vi "setControlTargetRange.vi"(8 "error":errorcluster, 9 "range":i32, 10 "axis":i32, 11 "connection ID":refnum<k5>) -> (0 "error out":errorcluster, 2 "axis_out":i32, 3 "connection ID out":refnum<k5>)   [LabVIEW 2016, in "amc_api.lvlib"]
doc: "This function sets the range around the target position in which the flag \"In Target Range\" (see VIII.7.a) becomes active."
uses:
  amc_api.lvlib
panel:
  out "jsonRespIn":string
  out "JSON-response":string="{\"jsonrpc\":\"2.0\",\"method\":\"\",\"params\":[5,1.245,true,\"name\"],\"id\":\"1\"}"
  out "JSON request":string
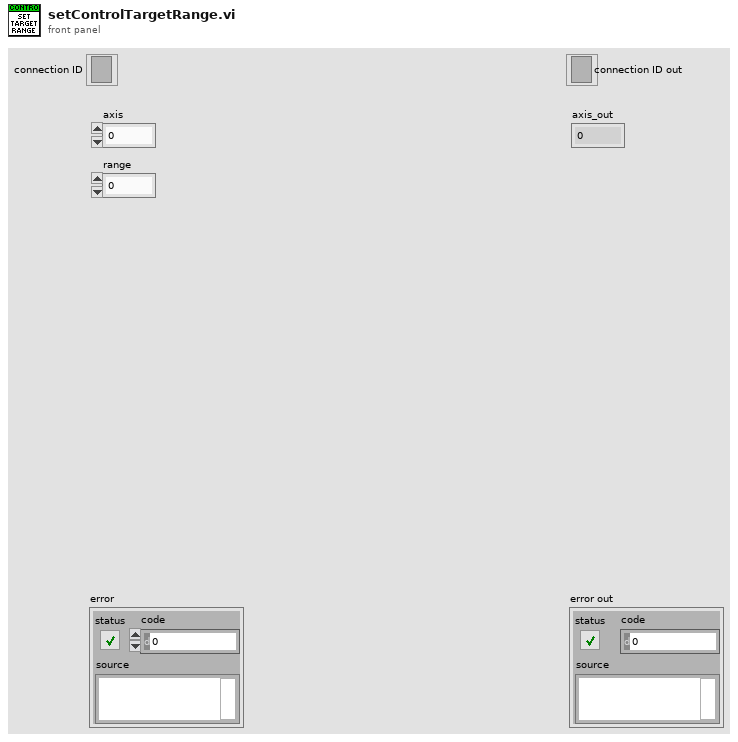
[diagram p1: front panel]
types:
  T1 = cluster{"jsonrpc":string, "method":string, "params":string[], "id":string, "api":i32, "pid":string}
  T2 = enum16{"Standard", "Buffered", "CRLF", "Immediate"}
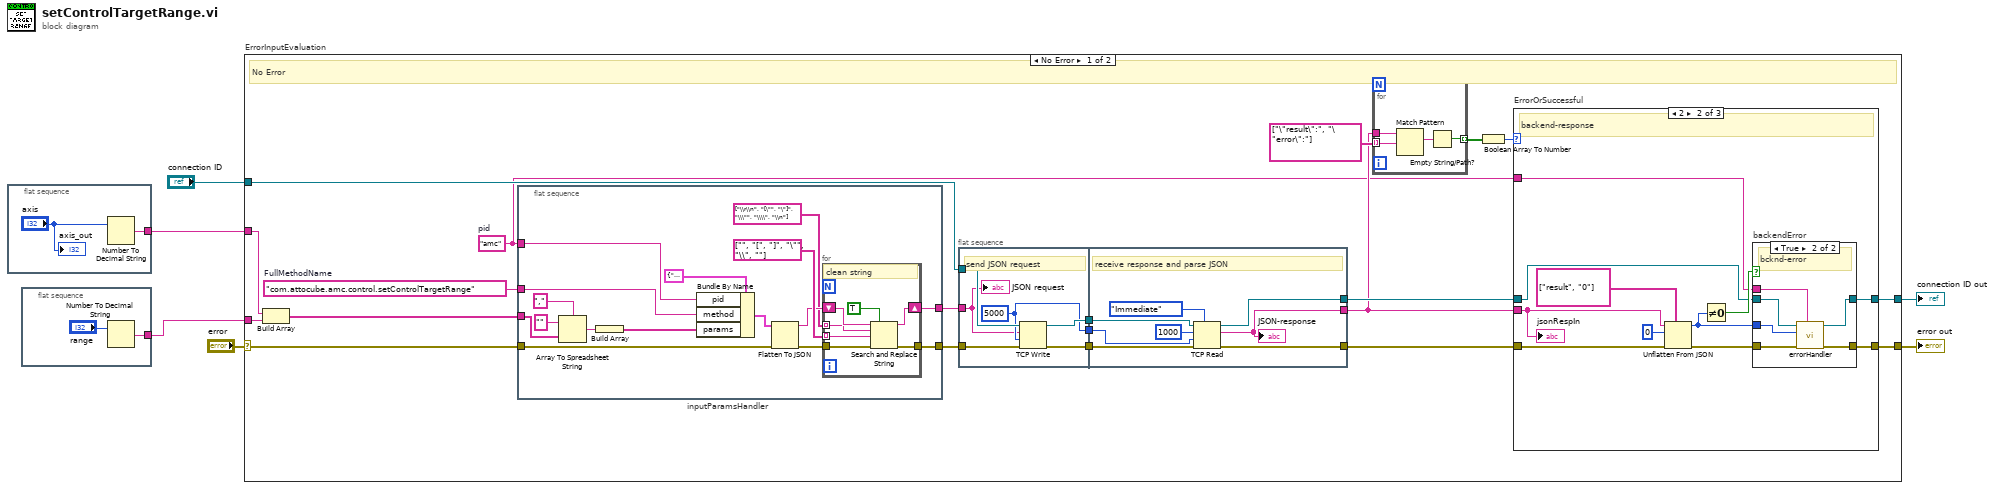
[diagram p0: block diagram]
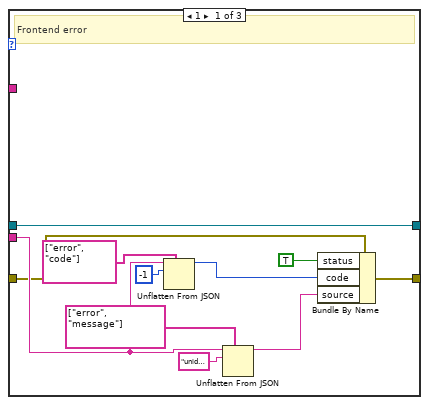
[diagram p2: hidden frame]
diagram:
  n1 = flat-sequence "in_axis" {
    tunnel: [w8] -> w2
    frame #0 {
      n2 = Number To Decimal String(number="axis") -> (decimal integer string=w8:string)  [unwired: 1 in]
      "axis_out" <- "axis"
    }
  }
  n3 = flat-sequence "in_integer" {
    tunnel: [w9] -> w1
    frame #0 {
      n4 = Number To Decimal String(number="range") -> (decimal integer string=w9:string)  [unwired: 1 in]
    }
  }
  n5 = case "ErrorInputEvaluation" shown="No Error" "error" {
    selector: "error" -> [w17 w104]
    tunnel: "connection ID" -> [w27 w105]
    tunnel: [w19 w104] -> w5
    tunnel: [w20 w105] -> w4
    tunnel: w2 -> [w12 _]
    tunnel: w1 -> [w11 _]
    frame No Error {
      w13 = "amc"  # pid
      w18 = "com.attocube.amc.control.setControlTargetRange"  # FullMethodName
      # "No Error"
      n6 = Build Array ("ParametersArrayString")(w12, w11) -> (w16:string[])
      n7 = flat-sequence "inputParamsHandler" {
        tunnel: [w36] -> w15
        tunnel: w16 -> [w42]
        tunnel: w17 -> [w41]
        tunnel: [w38] -> w14
        tunnel: w18 -> [w32]
        tunnel: w13 -> [w31]
        frame #0 {
          n8 = Array To Spreadsheet String(delimiter (Tab)=",", array=w42, 3:"" ("format string")) -> (spreadsheet string=w44:string)
          n9 = Build Array "Build Array"(w44) -> (w33:string[])
          n10 = Bundle By Name(cluster=T1 {"jsonrpc"="2.0", "method"="com.attocube.amc.res.setRESReadOutFreq", "params"=[], "id"="1", "api"=2, "pid"=""}, "pid"=w31, "method"=w32, "params"=w33) -> (w43:T1)
          n11 = Flatten To JSON(anything=w43, error in (no error)=w41) -> (JSON string=w37:string, 11:w39:errorcluster)  [unwired: 1 in]
          n12 = for {
            tunnel: string[] ["\\r\\n", "[\"", "\"]", "\\\"", "\\\\", "\\n"] ("search string") -> [w50] mode=indexing
            tunnel: string[] ["", "[", "]", "\"", "\\", ""] ("replace string (\"\")") -> [w49] mode=indexing
            shift-right: [w52] -> w36
            shift-left: w37 -> [w51]
            tunnel: w39 -> [w48]
            tunnel: [w47] -> w38
            # "clean string"
            n13 = Search and Replace String(replace all?=TRUE ("replace all? (F)"), input string=w51, search string=w50, replace string=w49, error in=w48) -> (result string=w52:string, error out=w47:errorcluster)  [unwired: 3 in, 2 out]
          }
        }
      }
      n14 = flat-sequence {
        tunnel: w27 -> [w95]
        tunnel: [w93] -> w30
        tunnel: [w94] -> w29
        tunnel: w14 -> [w90]
        tunnel: [w92] -> w28
        tunnel: w15 -> [w91]
        tunnel: [w99] -> w23
        tunnel: w30 -> [w101]
        tunnel: w29 -> [w100]
        tunnel: [w97] -> w22
        tunnel: w28 -> [w98]
        tunnel: [w96] -> w21
        frame #0 {
          w92 = 5000 ("timeout ms (25000)")
          # "send JSON request"
          n15 = TCP Write(connection ID=w95, data in=w91, error in (no error)=w90, 9:w92) -> (connection ID out=w93:refnum<k5>, error out=w94:errorcluster)  [unwired: 1 out]
          "JSON request" <- w91
        }
        frame #1 {
          # "receive response and parse JSON"
          n16 = TCP Read(connection ID=w101, bytes to read=1000, error in (no error)=w100, 7:T2."Immediate" ("mode (standard)"), 9:w98) -> (connection ID out=w99:refnum<k5>, data out=w96:string, error out=w97:errorcluster)
          "JSON-response" <- w96
        }
      }
      n17 = for {
        tunnel: string[] ["\"result\":", "\"error\":"] ("path") -> [w56] mode=indexing
        tunnel: [w54] -> w25 mode=indexing
        tunnel: w21 -> [w57]
        n18 = Match Pattern(string=w57, regular expression=w56) -> (match substring=w55:string)  [unwired: 1 in, 3 out]
        n19 = Empty String/Path?(string/path=w55) -> (empty?=w54:bool)
      }
      n20 = Boolean Array To Number(Boolean array=w25) -> (number=w24:u32)
      n21 = case "ErrorOrSuccessful" shown="2" w24 {
        tunnel: w21 -> [w60 w70 _]
        tunnel: w23 -> [w58 w73 w89]
        tunnel: [w58 w72 w89] -> w20
        tunnel: [w61 w71 w88] -> w19
        tunnel: w22 -> [w59 w74 w88]
        tunnel: w13 -> [_ w69 _]
        frame 1 {
          # "Frontend error"
          n22 = Unflatten From JSON(path=string[] ["error", "code"], JSON string=w60, type and defaults=-1) -> (value=w67:i32)  [unwired: 4 in, 1 out]
          n23 = Unflatten From JSON(path=string[] ["error", "message"], JSON string=w60, type and defaults="unidentified error") -> (value=w68:string)  [unwired: 4 in, 1 out]
          n24 = Bundle By Name(cluster=w59, "status"=TRUE, "code"=w67, "source"=w68) -> (w61:errorcluster)
        }
        frame 2 {
          # "backend-response"
          n25 = Unflatten From JSON(path=string[] ["result", "0"], JSON string=w70, type and defaults=0, error in (no error)=w74) -> (value=w79:i32, error out=w77:errorcluster)  [unwired: 3 in]
          n26 = Not Equal To 0?(x=w79) -> (x != 0?=w78:bool)
          n27 = case "backendError" shown="True" w78 {
            tunnel: w79 -> [_ w87]
            tunnel: w77 -> [w81 w86]
            tunnel: [w80 w85] -> w72
            tunnel: [w81 w84] -> w71
            tunnel: w73 -> [w80 w83]
            tunnel: w69 -> [_ w82]
            frame False {
              # "successful"
            }
            frame True {
              # "bcknd-error"
              n28 = call "errorHandler.vi"("pid"=w82, "error in"=w86, "errNbr"=w87, "connection ID"=w83) -> ("error out 2"=w84:errorcluster, "connection ID out"=w85:refnum<k5>)  [unwired: 6 in]
            }
          }
          "jsonRespIn" <- w70
        }
        frame Default {
          # "NoResponse"
        }
      }
    }
    frame Error {
      # "Error"
    }
  }
  "error out" <- w5
  "connection ID out" <- w4
